vi "按时间和编号查询.vi"(6 "结束时间":timestamp, 9 "起始时间":timestamp, 10 "回放吊点号":string, 11 "自动化引用句柄输入":refnum<k7>) -> (2 "位移":dbl[](array[numeric]), 3 "载荷":dbl[](array[numeric]))   [LabVIEW 2018]
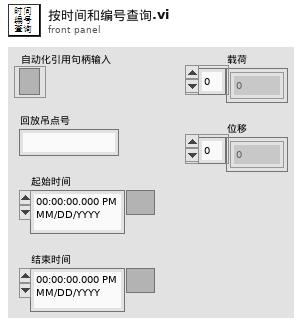
[diagram p1: front panel]
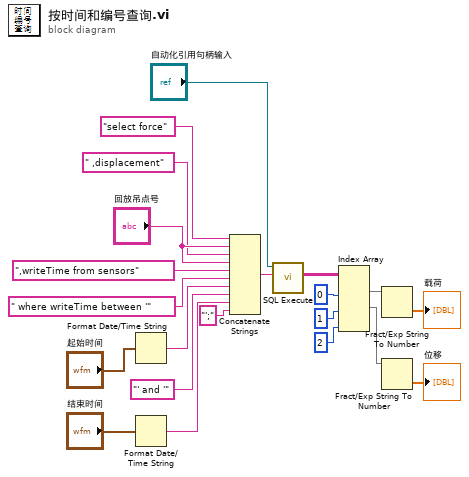
[diagram p0: block diagram]
diagram:
  n1 = Format Date/Time String(seconds (now)="起始时间") -> (date/time string=w7:string)  [unwired: 2 in]
  n2 = Format Date/Time String(seconds (now)="结束时间") -> (date/time string=w9:string)  [unwired: 2 in]
  n3 = Concatenate Strings("select force" ("字符串"), "回放吊点号", " ,displacement" ("字符串"), "回放吊点号", ",writeTime from sensors" ("Command Text"), " where writeTime between '" ("字符串"), w7, "' and '" ("字符串"), w9, "';" ("字符串")) -> (w11:string)
  n4 = call <userlib>:"SQL Execute.vi"("Command Text"=w11, "ADODB._Connection In"="自动化引用句柄输入") -> ("Data"=w15:string[][])  [unwired: 6 in, 3 out]
  n5 = Index Array(array=w15, index (col) #1=0 ("禁用的索引 (列)"), index (col) #2=1 ("索引 (列)"), index (col) #3=2 ("索引 (列)")) -> (element #1=w18:string[], element #2=w20:string[])  [unwired: 3 in, 1 out]
  n6 = Fract/Exp String To Number(string=w18) -> (number=→"载荷":dbl[])  [unwired: 3 in, 1 out]
  n7 = Fract/Exp String To Number(string=w20) -> (number=→"位移":dbl[])  [unwired: 3 in, 1 out]
